vi "Register gRPC Messages.vi"(8 "error in (no error)":errorcluster, 10 "package":string, 11 "gRPC ID":T1) -> (0 "error out":errorcluster, 3 "gRPC ID Out":T1)   [LabVIEW 2019, in "MicronGRPCGeneratedClient.lvlib"]
uses:
  MicronGRPCGeneratedClient.lvlib
  <vilib>/gRPC/LabVIEW gRPC Library/grpc-lvsupport-release.lvlib
  <vilib>/gRPC/LabVIEW gRPC Library/Server API/typeDefs/Message Metadata.ctl
  <vilib>/gRPC/LabVIEW gRPC Library/Server API/typeDefs/Message Element Type.ctl
  <vilib>/gRPC/LabVIEW gRPC Library/Server API/typeDefs/Message Element Metadata.ctl
  <vilib>/gRPC/LabVIEW gRPC Library/Server API/typeDefs/Enum Metadata.ctl
  <vilib>/SLL Toolkit/SLL String/SLL String.lvlib
  <vilib>/gRPC/LabVIEW gRPC Library/Shared/grpcId.ctl
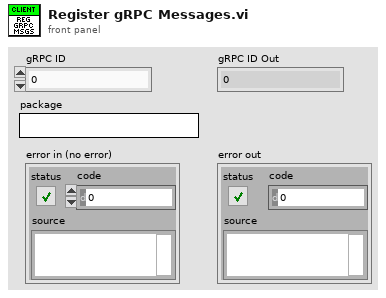
[diagram p1: front panel]
types:
  T1 = typedef "grpc-lvsupport-release.lvlib/grpcId.ctl" = u64
  T2 = typedef "grpc-lvsupport-release.lvlib/Enum Metadata.ctl" = cluster{"Version":i32, "Name":string, "Type Url":string, "Enum Values":string, "Allow Alias":bool}
  T3 = typedef "grpc-lvsupport-release.lvlib/Message Metadata.ctl" = cluster{"Version":i32, "Name":string, "Type Url":string, "Elements":T4[], "Has Oneof":bool}
  T4 = typedef "grpc-lvsupport-release.lvlib/Message Element Metadata.ctl" = cluster{"Field Name":string, "Embedded Message Name":string, "Protobuf Index":i32, "MessageElementType":T5, "Repeated":bool, "Is in Oneof":bool, "Oneof Container Name":string}
  T5 = typedef "grpc-lvsupport-release.lvlib/Message Element Type.ctl" = enum32{"Int32Value", "FloatValue", "DoubleValue", "BoolValue", "StringValue", "MessageValue", "Int64Value", "UInt32Value", "UInt64Value", "EnumValue", "Bytes", "Fixed64", "Fixed32", "SFixed64", "SFixed32", "SInt64", "SInt32"}
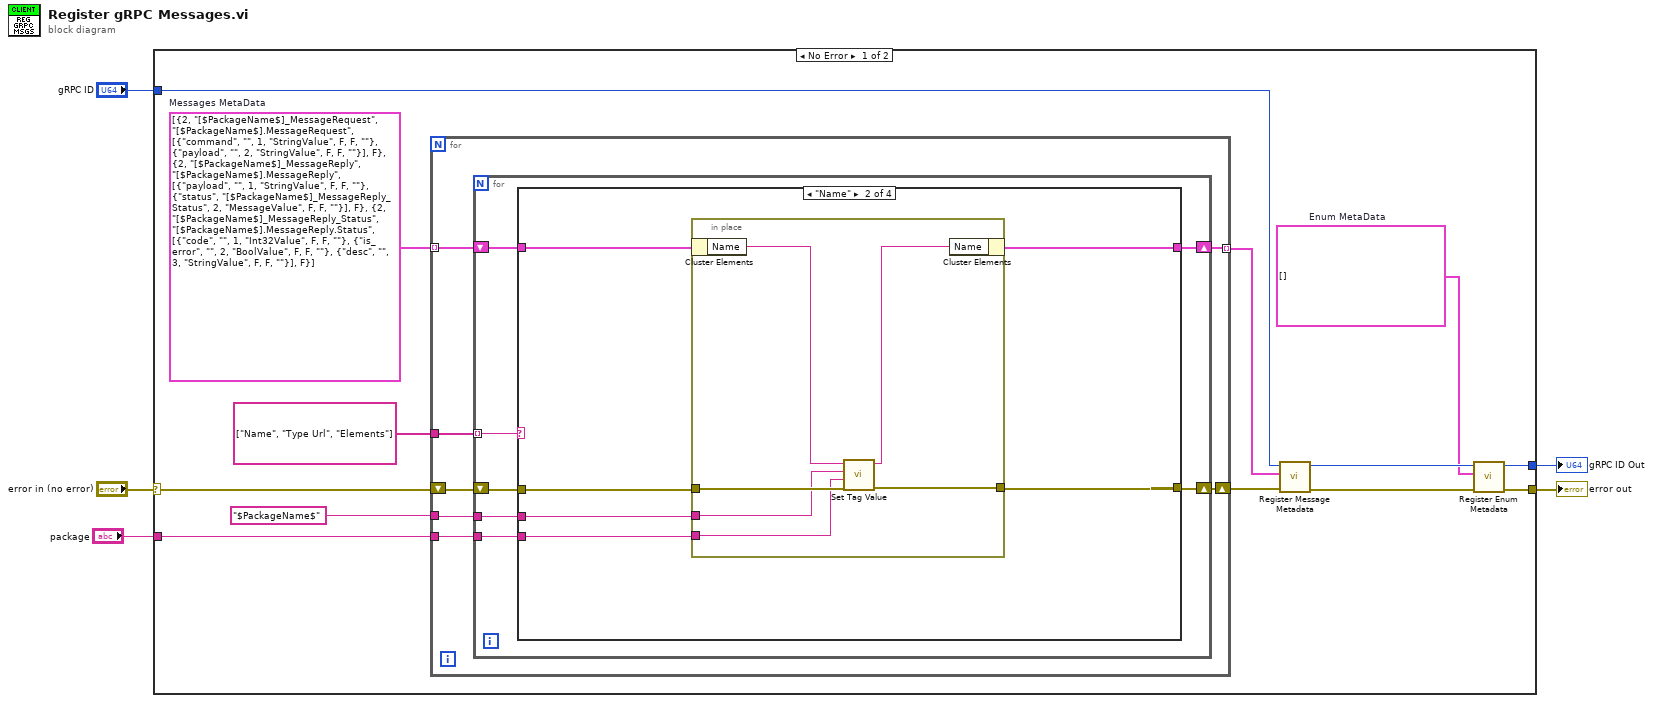
[diagram p0: block diagram]
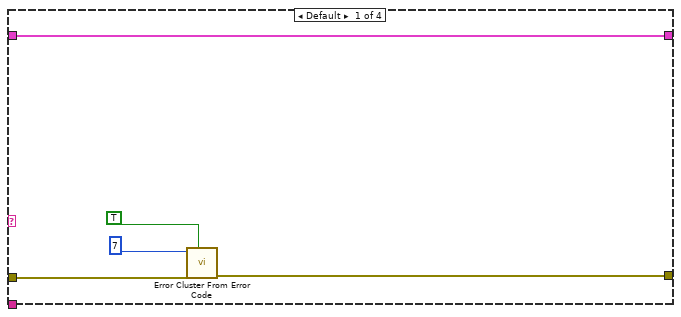
[diagram p2: hidden frame]
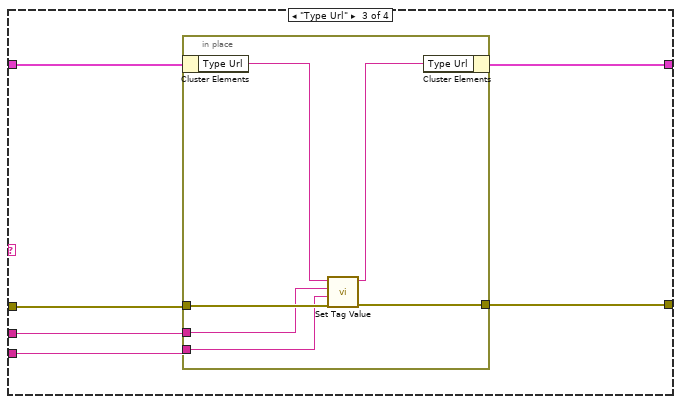
[diagram p3: hidden frame]
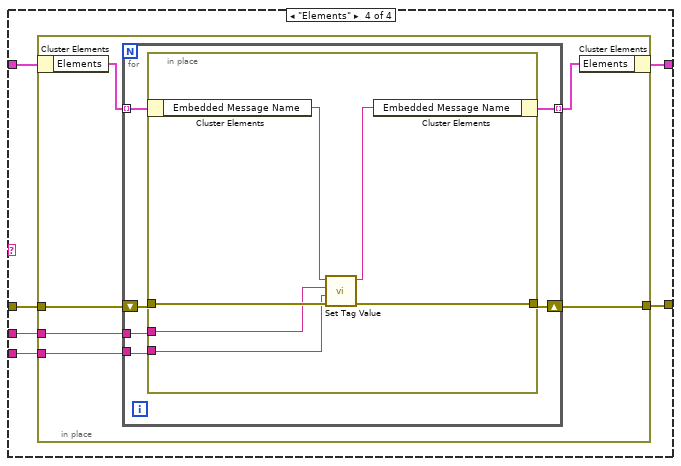
[diagram p4: hidden frame]
diagram:
  n1 = case shown="No Error" "error in (no error)" {
    selector: "error in (no error)" -> [w10 w86]
    tunnel: [w17 w85] -> w2
    tunnel: [w14 w86] -> w5
    tunnel: "gRPC ID" -> [w17 w85]
    tunnel: "package" -> [w8 _]
    frame No Error {
      w13 = T2[] []  # Enum MetaData
      w11 = T3[] [{"Version"=2, "Name"="[$PackageName$]_MessageRequest", "Type Url"="[$PackageName$].MessageRequest", "Elements"=[{"Field Name"="command", "Embedded Message Name"="", "Protobuf Index"=1, "MessageElementType"=enum."StringValue", "Repeated"=FALSE, "Is in Oneof"=FALSE, "Oneof Container Name"=""}, {"Field Name"="payload", "Embedded Message Name"="", "Protobuf Index"=2, "MessageElementType"=enum."StringValue", "Repeated"=FALSE, "Is in Oneof"=FALSE, "Oneof Container Name"=""}], "Has Oneof"=FALSE}, {"Version"=2, "Name"="[$PackageName$]_MessageReply", "Type Url"="[$PackageName$].MessageReply", "Elements"=[{"Field Name"="payload", "Embedded Message Name"="", "Protobuf Index"=1, "MessageElementType"=enum."StringValue", "Repeated"=FALSE, "Is in Oneof"=FALSE, "Oneof Container Name"=""}, {"Field Name"="status", "Embedded Message Name"="[$PackageName$]_MessageReply_Status", "Protobuf Index"=2, "MessageElementType"=enum."MessageValue", "Repeated"=FALSE, "Is in Oneof"=FALSE, "Oneof Container Name"=""}], "Has Oneof"=FALSE}, {"Version"=2, "Name"="[$PackageName$]_MessageReply_Status", "Type Url"="[$PackageName$].MessageReply.Status", "Elements"=[{"Field Name"="code", "Embedded Message Name"="", "Protobuf Index"=1, "MessageElementType"=enum."Int32Value", "Repeated"=FALSE, "Is in Oneof"=FALSE, "Oneof Container Name"=""}, {"Field Name"="is_error", "Embedded Message Name"="", "Protobuf Index"=2, "MessageElementType"=enum."BoolValue", "Repeated"=FALSE, "Is in Oneof"=FALSE, "Oneof Container Name"=""}, {"Field Name"="desc", "Embedded Message Name"="", "Protobuf Index"=3, "MessageElementType"=enum."StringValue", "Repeated"=FALSE, "Is in Oneof"=FALSE, "Oneof Container Name"=""}], "Has Oneof"=FALSE}]  # Messages MetaData
      n2 = for {
        tunnel: [w18] -> w12 mode=indexing
        tunnel: w11 -> [w22] mode=indexing
        tunnel: "$PackageName$" ("Tag Name") -> [w21]
        tunnel: w8 -> [w23]
        tunnel: string[] ["Name", "Type Url", "Elements"] -> [w20]
        shift-right: [w19] -> w6
        shift-left: w10 -> [w24]
        n3 = for {
          tunnel: w23 -> [w30]
          tunnel: w21 -> [w28]
          tunnel: w20 -> [w27] mode=indexing
          shift-right: [w26] -> w19
          shift-left: w24 -> [w31]
          shift-right: [w25] -> w18
          shift-left: w22 -> [w29]
          n4 = case shown="\"Name\"" w27 {
            tunnel: w31 -> [w36 w42 w54 w66]
            tunnel: w30 -> [_ w41 w53 w65]
            tunnel: w29 -> [w32 w40 w52 w64]
            tunnel: w28 -> [_ w39 w51 w63]
            tunnel: [w33 w37 w49 w61] -> w26
            tunnel: [w32 w38 w50 w62] -> w25
            frame Default {
              n5 = call <vilib>:"Error Cluster From Error Code.vi"("show call chain? (False)"=TRUE, "error in (no error)"=w36, "error code (0)"=7) -> ("error out"=w33:errorcluster)  [unwired: 6 in]
            }
            frame "Name" {
              n6 = in-place {
                in-place-border: w42 -> [w48]
                in-place-border: w39 -> [w44]
                in-place-border: w41 -> [w43]
                in-place-border: [w45] -> w37
                n7 = in-place-cluster #1(w40) -> ("Name"=w47:string)
                n8 = call <vilib>:"Set Tag Value.vi"("error in (no error)"=w48, "Tag Value"=w43, "Tag Name"=w44, "Input String"=w47) -> ("error out"=w45:errorcluster, "Output String"=w46:string)  [unwired: 6 in]
                n9 = in-place-cluster #1("Name"=w46) -> (w38:T3)
              }
            }
            frame "Type Url" {
              n10 = in-place {
                in-place-border: w54 -> [w60]
                in-place-border: w51 -> [w56]
                in-place-border: w53 -> [w55]
                in-place-border: [w57] -> w49
                n11 = in-place-cluster #2(w52) -> ("Type Url"=w59:string)
                n12 = call <vilib>:"Set Tag Value.vi"("error in (no error)"=w60, "Tag Value"=w55, "Tag Name"=w56, "Input String"=w59) -> ("error out"=w57:errorcluster, "Output String"=w58:string)  [unwired: 6 in]
                n13 = in-place-cluster #2("Type Url"=w58) -> (w50:T3)
              }
            }
            frame "Elements" {
              n14 = in-place {
                in-place-border: w66 -> [w72]
                in-place-border: w63 -> [w70]
                in-place-border: w65 -> [w69]
                in-place-border: [w71] -> w61
                n15 = in-place-cluster #3(w64) -> ("Elements"=w68:T4[])
                n16 = for {
                  tunnel: w70 -> [w76]
                  tunnel: w69 -> [w75]
                  shift-right: [w77] -> w71
                  shift-left: w72 -> [w78]
                  tunnel: w68 -> [w74] mode=indexing
                  tunnel: [w73] -> w67 mode=indexing
                  n17 = in-place {
                    in-place-border: w78 -> [w84]
                    in-place-border: [w83] -> w77
                    in-place-border: w76 -> [w82]
                    in-place-border: w75 -> [w81]
                    n18 = in-place-cluster #4(w74) -> ("Embedded Message Name"=w80:string)
                    n19 = call <vilib>:"Set Tag Value.vi"("error in (no error)"=w84, "Tag Value"=w81, "Tag Name"=w82, "Input String"=w80) -> ("error out"=w83:errorcluster, "Output String"=w79:string)  [unwired: 6 in]
                    n20 = in-place-cluster #4("Embedded Message Name"=w79) -> (w73:T4)
                  }
                }
                n21 = in-place-cluster #3("Elements"=w67) -> (w62:T3)
              }
            }
          }
        }
      }
      n22 = call <vilib>:"Register Message Metadata.vi"("error in"=w6, "Messages"=w12, "gRPCid in"=w17) -> ("error out"=w15:errorcluster, "gRPCid out"=w16:T1)  [unwired: 7 in]
      n23 = call <vilib>:"Register Enum Metadata.vi"("error in"=w15, "Enum Metadata"=w13, "gRPCid in"=w16) -> ("error out"=w14:errorcluster)  [unwired: 7 in, 1 out]
    }
    frame Error {
    }
  }
  "error out" <- w5
  "gRPC ID Out" <- w2
